vi "To Generic.vi"(8 "error in (no error)":errorcluster, 11 "Instrument Error Data in":refnum<class "Instrument Error Data.lvclass">) -> (0 "error out":errorcluster, 2 "Generic Data":refnum<class "Generic Data.lvclass">[](array[class]), 3 "Data Name":string[](array[string]))   [LabVIEW 2020, in "Instrument Handler.lvlib" / "Instrument Error Data.lvclass"]
doc: "Present private data as an array of named generic data elements."
uses:
  Instrument Error Data.lvclass
  PPL/HDH.Data.Generic.lvlibp/Generic Data/Generic Data.lvclass
  Instrument Error Data.lvclass/Instrument Error Data.ctl
  PPL/HDH.Data.Generic.lvlibp/Generic Data/Time Stamp/Time Stamp.lvclass
  C:/Current projects/WS/PPL/HDH.Data.Generic.lvlibp/Generic Data/Generic Data.lvclass
  PPL/HDH.Data.Generic.lvlibp/Generic Data/String/String.lvclass
  PPL/HDH.Data.Generic.lvlibp/Generic Data/I32/I32.lvclass
  PPL/HDH.Data.Generic.lvlibp/Data.lvclass
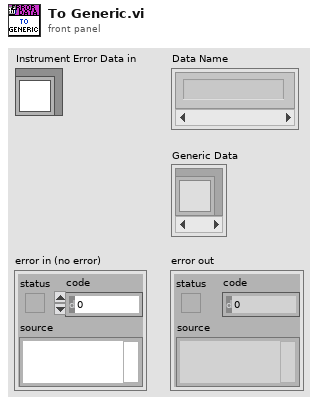
[diagram p1: front panel]
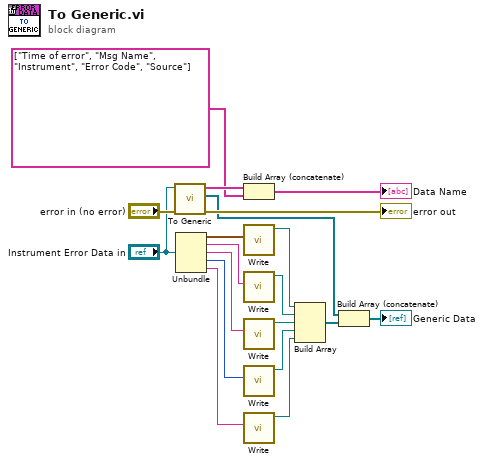
[diagram p0: block diagram]
diagram:
  n1 = call-parent "To Generic.vi"("error in (no error)"="error in (no error)", "Data in"="Instrument Error Data in") -> ("error out"=→"error out":errorcluster, "Generic Data"=w11:refnum<class "Generic Data.lvclass">[], "Data Name"=w16:string[])  [unwired: 7 in]
  n2 = Unbundle("Instrument Error Data in") -> (w13:timestamp, w8:string, w6:string, w4:i32, w2:string)
  n3 = Build Array (concatenate)(w16, string[] ["Time of error", "Msg Name", "Instrument", "Error Code", "Source"] ("array")) -> (→"Data Name":string[])
  n4 = call "Write.vi"("Time Stamp"=w13) -> ("Time Stamp out"=w12:refnum<class "Time Stamp.lvclass">)  [unwired: 10 in]
  n5 = call "Write.vi"("String"=w8) -> ("String out"=w7:refnum<class "String.lvclass">)  [unwired: 10 in]
  n6 = call "Write.vi"("String"=w6) -> ("String out"=w5:refnum<class "String.lvclass">)  [unwired: 10 in]
  n7 = call "Write.vi"("I32"=w4) -> ("I32 out"=w3:refnum<class "I32.lvclass">)  [unwired: 10 in]
  n8 = call "Write.vi"("String"=w2) -> ("String out"=w1:refnum<class "String.lvclass">)  [unwired: 10 in]
  n9 = Build Array(w12, w7, w5, w3, w1) -> (w10:refnum<class "Generic Data.lvclass">[])
  n10 = Build Array (concatenate)(w11, w10) -> (→"Generic Data":refnum<class "Generic Data.lvclass">[])
